vi "zwangstest.vi"() -> ()   [LabVIEW 2010]
panel:
  in  "Stopp 2":bool
  out "Zwangsbedingung!":dbl[](array[numeric])
  out "Zwangsbedingung?":bool[](array[boolean])
  in  "AbfragbVariablen":dbl[](array[numeric])
  out "Zwangsneurosen":string[][](array[string])
  in  "Bedingung Nr. X":i32
  in  "löschen":bool
  in  "Bedingung übernehmen":bool
  in  "Stopp":bool
  in  "Wert 2":dbl
  in  "Wert 1":dbl
  in  "Vergleichsoperator":dbl(ring) items=["<", "<=", "=", ">=", ">", "=/="]
  in  "BedienbareVariablen":dbl(ring) items=["Mod5/DIO0", "Mod5/DIO1", "Mod5/DIO2", "Mod5/DIO3", "Mod5/DIO4", "Mod5/DIO5", "Mod5/DIO6", "Mod5/DIO7", "Mod5/DIO8", "Mod5/DIO9", "Mod5/DIO10", "Mod5/DIO11", "Mod5/DIO12", "Mod5/DIO13", "Mod5/DIO14", "Mod5/DIO15", "Mod5/DIO16", "Mod5/DIO17", "Mod5/DIO18", "Mod5/DIO19", "Mod5/DIO20", "Mod5/DIO21", "Mod5/DIO22", "Mod5/DIO23", "Mod5/DIO24", "Mod5/DIO25", "Mod5/DIO26", "Mod5/DIO27", "Mod5/DIO28", "Mod5/DIO29", "Mod5/DIO30", "Mod5/DIO31", "Mod6/DIO0", "Mod6/DIO1", "Mod6/DIO2", "Mod6/DIO3", "Mod6/DIO4", "Mod6/DIO5", "Mod6/DIO6", "Mod6/DIO7", "Mod6/DIO8", "Mod6/DIO9", "Mod6/DIO10", "Mod6/DIO11", "Mod6/DIO12", "Mod6/DIO13", "Mod6/DIO14", "Mod6/DIO15", "Mod6/DIO16", "Mod6/DIO17", "Mod6/DIO18", "Mod6/DIO19", "Mod6/DIO20", "Mod6/DIO21", "Mod6/DIO22", "Mod6/DIO23", "Mod6/DIO24", "Mod6/DIO25", "Mod6/DIO26", "Mod6/DIO27", "Mod6/DIO28", "Mod6/DIO29", "Mod6/DIO30", "Mod6/DIO31", "ServoTrap1kalt", "ServoTrap2kalt", "Heizen?Trap1", "Heizen?Trap2", "Heizen?Mach1", "Heizen?Mach2", "LHHorst1Heizen?", "LHMainCol1Heizen?", "LHMainCol2Heizen?", "LHHorst2Heizen?", "LHOvenHeizen?", "LHT-LineHeizen?", "SPHorst1", "SPHorst2", "SPHorst3", "SPHorst4", "SPHorst5", "SPHorst6", "SPHorst7", "SPHorst8", "SPHorst9", "SPHorst10", "SPHorst11", "SPHorst12", "SPHorst13", "SPHorst14", "SPHorst15"]
  in  "AbfragbareVariablen":dbl(ring) items=["Mod1/AI0", "Mod1/AI1", "Mod1/AI2", "Mod1/AI3", "Mod1/AI4", "Mod1/AI5", "Mod1/AI6", "Mod1/AI7", "Mod1/AI8", "Mod1/AI9", "Mod1/AI10", "Mod1/AI11", "Mod1/AI12", "Mod1/AI13", "Mod1/AI14", "Mod1/AI15", "Mod1/AI16", "Mod1/AI17", "Mod1/AI18", "Mod1/AI19", "Mod1/AI20", "Mod1/AI21", "Mod1/AI22", "Mod1/AI23", "Mod1/AI24", "Mod1/AI25", "Mod1/AI26", "Mod1/AI27", "Mod1/AI28", "Mod1/AI29", "Mod1/AI30", "Mod1/AI31", "Mod2/AI0", "Mod2/AI1", "Mod2/AI2", "Mod2/AI3", "Mod2/AI4", "Mod2/AI5", "Mod2/AI6", "Mod2/AI7", "Mod2/AI8", "Mod2/AI9", "Mod2/AI10", "Mod2/AI11", "Mod2/AI12", "Mod2/AI13", "Mod2/AI14", "Mod2/AI15", "Mod2/AI16", "Mod2/AI17", "Mod2/AI18", "Mod2/AI19", "Mod2/AI20", "Mod2/AI21", "Mod2/AI22", "Mod2/AI23", "Mod2/AI24", "Mod2/AI25", "Mod2/AI26", "Mod2/AI27", "Mod2/AI28", "Mod2/AI29", "Mod2/AI30", "Mod2/AI31", "Mod3/AI0", "Mod3/AI1", "Mod3/AI2", "Mod3/AI3", "Mod3/AI4", "Mod3/AI5", "Mod3/AI6", "Mod3/AI7", "Mod3/AI8", "Mod3/AI9", "Mod3/AI10", "Mod3/AI11", "Mod3/AI12", "Mod3/AI13", "Mod3/AI14", "Mod3/AI15", "Mod3/AI16", "Mod3/AI17", "Mod3/AI18", "Mod3/AI19", "Mod3/AI20", "Mod3/AI21", "Mod3/AI22", "Mod3/AI23", "Mod3/AI24", "Mod3/AI25", "Mod3/AI26", "Mod3/AI27", "Mod3/AI28", "Mod3/AI29", "Mod3/AI30", "Mod3/AI31", "WiderstTrap1", "TempTrap1", "WiderstTrap2", "TempTrap2", "TempMach1", "TempMach2", "MWHorst1", "MWHorst2", "MWHorst3", "MWHorst4", "MWHorst5", "MWHorst6", "MWHorst7", "MWHorst8", "MWHorst9", "MWHorst10", "MWHorst11", "MWHorst12", "MWHorst13", "MWHorst14", "MWHorst15"]
  # "===>>"
  # "="
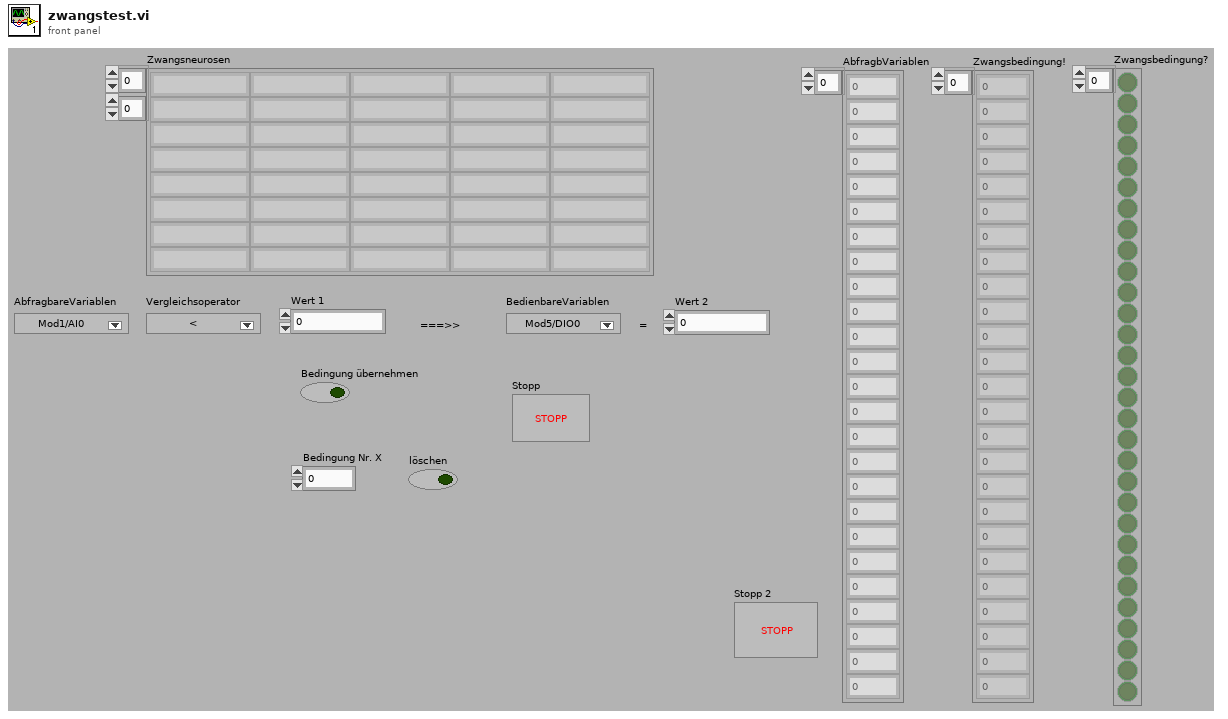
[diagram p1: front panel]
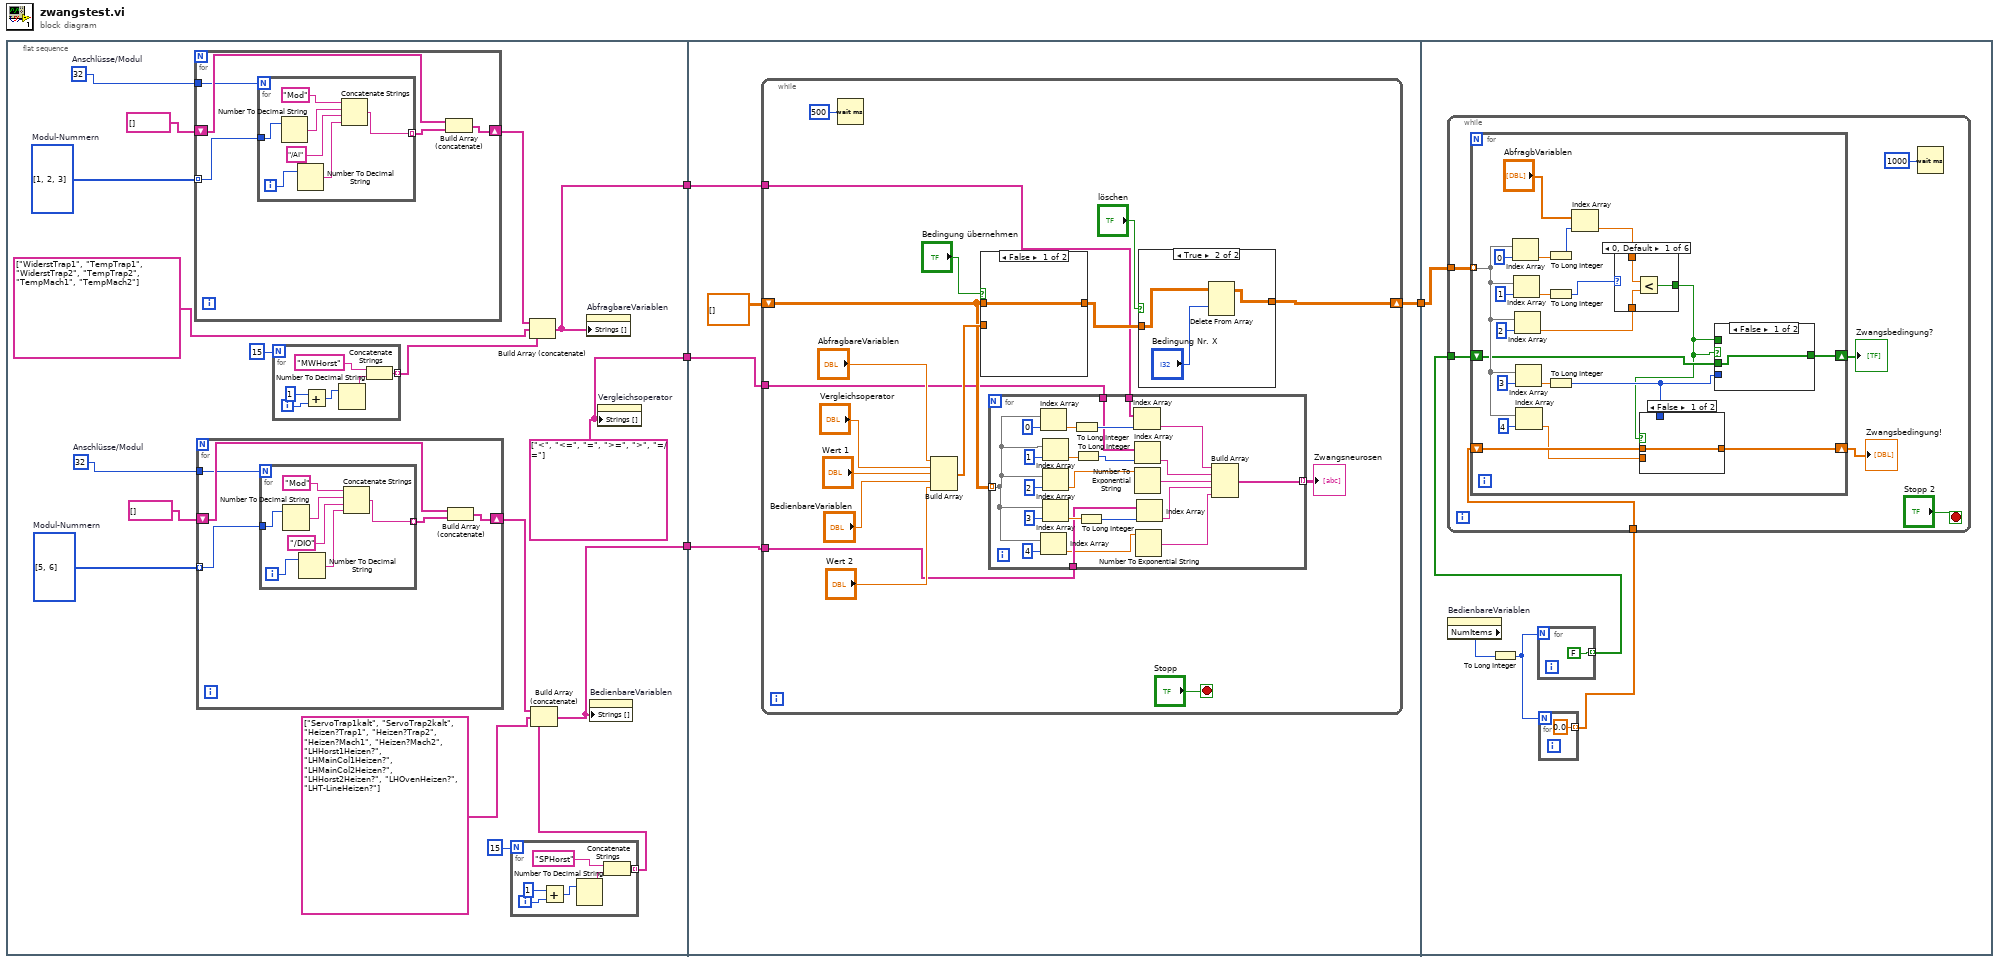
[diagram p0: block diagram]
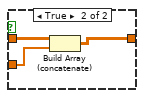
[diagram p3: hidden frame]
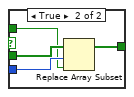
[diagram p4: hidden frame]
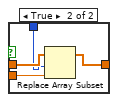
[diagram p5: hidden frame]
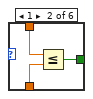
[diagram p6: hidden frame]
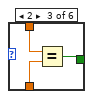
[diagram p7: hidden frame]
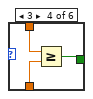
[diagram p8: hidden frame]
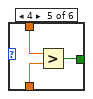
[diagram p9: hidden frame]
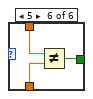
[diagram p10: hidden frame]
diagram:
  n1 = flat-sequence {
    tunnel: [w13] -> w4
    tunnel: [w12] -> w3
    tunnel: [w11] -> w2
    tunnel: w4 -> [w61]
    tunnel: w3 -> [w60]
    tunnel: w2 -> [w59]
    tunnel: [w58] -> w1
    tunnel: w1 -> [w112]
    frame #0 {
      w12 = string[] ["<", "<=", "=", ">=", ">", "=/="] ("Strings []")
      w16 = 32  # Anschlüsse/Modul
      w15 = i32[] [5, 6]  # Modul-Nummern
      w20 = 32  # Anschlüsse/Modul
      w19 = i32[] [1, 2, 3]  # Modul-Nummern
      n2 = for {
        shift-right: [w48] -> w21
        shift-left: string[] [] -> [w50]
        tunnel: w19 -> [w47] mode=indexing
        tunnel: w20 -> [w46]
        n3 = for {
          N: w46 -> [_]
          tunnel: [w56] -> w49 mode=indexing
          tunnel: w47 -> [w54]
          i -> [w57]
          n4 = Number To Decimal String(number=w54) -> (decimal integer string=w53:string)  [unwired: 1 in]
          n5 = Number To Decimal String(number=w57) -> (decimal integer string=w51:string)  [unwired: 1 in]
          n6 = Concatenate Strings("Mod", w53, "/AI", w51) -> (w56:string)
        }
        n7 = Build Array (concatenate)(w50, w49) -> (w48:string[])
      }
      n8 = for {
        shift-right: [w36] -> w17
        shift-left: string[] [] -> [w38]
        tunnel: w15 -> [w35] mode=indexing
        tunnel: w16 -> [w34]
        n9 = for {
          N: w34 -> [_]
          tunnel: [w44] -> w37 mode=indexing
          tunnel: w35 -> [w42]
          i -> [w45]
          n10 = Number To Decimal String(number=w42) -> (decimal integer string=w41:string)  [unwired: 1 in]
          n11 = Number To Decimal String(number=w45) -> (decimal integer string=w39:string)  [unwired: 1 in]
          n12 = Concatenate Strings("Mod", w41, "/DIO", w39) -> (w44:string)
        }
        n13 = Build Array (concatenate)(w38, w37) -> (w36:string[])
      }
      n14 = for {
        N: 15 -> [_]
        tunnel: [w28] -> w7 mode=indexing
        i -> [w33]
        n15 = Add(x=1, y=w33) -> (x+y=w31:i32)
        n16 = Number To Decimal String(number=w31) -> (decimal integer string=w29:string)  [unwired: 1 in]
        n17 = Concatenate Strings("MWHorst", w29) -> (w28:string)
      }
      n18 = for {
        N: 15 -> [_]
        tunnel: [w22] -> w5 mode=indexing
        i -> [w27]
        n19 = Add(x=1, y=w27) -> (x+y=w25:i32)
        n20 = Number To Decimal String(number=w25) -> (decimal integer string=w23:string)  [unwired: 1 in]
        n21 = Concatenate Strings("SPHorst", w23) -> (w22:string)
      }
      n22 = Build Array (concatenate)(w21, string[] ["WiderstTrap1", "TempTrap1", "WiderstTrap2", "TempTrap2", "TempMach1", "TempMach2"], w7) -> (w13:string[])
      n23 = Build Array (concatenate)(w17, string[] ["ServoTrap1kalt", "ServoTrap2kalt", "Heizen?Trap1", "Heizen?Trap2", "Heizen?Mach1", "Heizen?Mach2", "LHHorst1Heizen?", "LHMainCol1Heizen?", "LHMainCol2Heizen?", "LHHorst2Heizen?", "LHOvenHeizen?", "LHT-LineHeizen?"], w5) -> (w11:string[])
      n24 = property on="AbfragbareVariablen" class="Ring (strikt)"("Strings []"=w13) -> ()  [unwired: 2 in, 2 out]
      n25 = property on="BedienbareVariablen" class="Ring (strikt)"("Strings []"=w11) -> ()  [unwired: 2 in, 2 out]
      n26 = property on="Vergleichsoperator" class="Ring (strikt)"("Strings []"=w12) -> ()  [unwired: 2 in, 2 out]
    }
    frame #1 {
      n27 = while {
        shift-right: [w69] -> w58
        shift-left: dbl[][] [] -> [w67]
        tunnel: w61 -> [w66]
        tunnel: w60 -> [w65]
        tunnel: w59 -> [w64]
        stop <- "Stopp" stop-if-true
        n28 = Wait (ms)(milliseconds to wait=u32 500 ("Zu wartende ms")) -> ()  [unwired: 1 out]
        n29 = Build Array("AbfragbareVariablen", "Vergleichsoperator", "Wert 1", "BedienbareVariablen", "Wert 2") -> (w71:dbl[])
        n30 = case shown="False" "Bedingung übernehmen" {
          tunnel: w67 -> [w107 w110]
          tunnel: w71 -> [_ w109]
          tunnel: [w107 w108] -> w70
          frame False {
          }
          frame True {
            n31 = Build Array (concatenate)(w110, w109) -> (w108:dbl[][])
          }
        }
        n32 = for {
          tunnel: w67 -> [w102] mode=indexing
          tunnel: w66 -> [w90]
          tunnel: w65 -> [w89]
          tunnel: w64 -> [w88]
          tunnel: [w80] -> w63 mode=indexing
          n33 = Index Array(array=w102, index=0 ("Index")) -> (element=w96:dbl)
          n34 = Index Array(array=w102, index=4 ("Index")) -> (element=w86:dbl)
          n35 = Index Array(array=w102, index=1 ("Index")) -> (element=w94:dbl)
          n36 = Index Array(array=w102, index=2 ("Index")) -> (element=w87:dbl)
          n37 = Index Array(array=w102, index=3 ("Index")) -> (element=w92:dbl)
          n38 = To Long Integer(number=w96) -> (32bit integer=w95:i32)
          n39 = To Long Integer(number=w94) -> (32bit integer=w93:i32)
          n40 = To Long Integer(number=w92) -> (32bit integer=w91:i32)
          n41 = Index Array(array=w90, index=w95) -> (element=w85:string)
          n42 = Index Array(array=w89, index=w93) -> (element=w84:string)
          n43 = Number To Exponential String(number=w87) -> (E-format string=w83:string)  [unwired: 3 in]
          n44 = Number To Exponential String(number=w86) -> (E-format string=w81:string)  [unwired: 3 in]
          n45 = Index Array(array=w88, index=w91) -> (element=w82:string)
          n46 = Build Array(w85, w84, w83, w82, w81) -> (w80:string[])
        }
        "Zwangsneurosen" <- w63
        n47 = case shown="True" "löschen" {
          tunnel: w70 -> [w103 w106]
          tunnel: [w103 w104] -> w69
          frame False {
          }
          frame True {
            n48 = Delete From Array(array=w106, index (row)="Bedingung Nr. X") -> (array with subset deleted=w104:dbl[][])  [unwired: 2 in, 1 out]
          }
        }
      }
    }
    frame #2 {
      n49 = property on="BedienbareVariablen" class="Ring (strikt)"() -> ("NumItems"=w114:u32)  [unwired: 2 in, 2 out]
      n50 = To Long Integer(number=w114) -> (32bit integer=w113:i32)
      n51 = for {
        N: w113 -> [_]
        tunnel: [FALSE] -> w115 mode=indexing
      }
      n52 = for {
        N: w113 -> [_]
        tunnel: [0.0] -> w111 mode=indexing
      }
      n53 = while {
        tunnel: w112 -> [w123]
        tunnel: w115 -> [w122]
        tunnel: w111 -> [w118]
        stop <- "Stopp 2" stop-if-true
        n54 = for {
          tunnel: w123 -> [w131] mode=indexing
          shift-right: [w124] -> w120
          shift-left: w122 -> [w127]
          shift-right: [w128] -> w117
          shift-left: w118 -> [w130]
          n55 = Index Array(array=w131, index=0 ("Index")) -> (element=w142:dbl)
          n56 = Index Array(array=w131, index=1 ("Index")) -> (element=w140:dbl)
          n57 = Index Array(array=w131, index=2 ("Index")) -> (element=w136:dbl)
          n58 = Index Array(array=w131, index=3 ("Index")) -> (element=w133:dbl)
          n59 = Index Array(array=w131, index=4 ("Index")) -> (element=w129:dbl)
          n60 = To Long Integer(number=w142) -> (32bit integer=w135:i32)
          n61 = To Long Integer(number=w140) -> (32bit integer=w139:i32)
          n62 = To Long Integer(number=w133) -> (32bit integer=w126:i32)
          n63 = Index Array(array="AbfragbVariablen", index=w135) -> (element=w138:dbl)
          n64 = case shown="0, Default" w139 {
            tunnel: w138 -> [w157 w159 w163 w166 w169 w172]
            tunnel: w136 -> [w156 w160 w162 w165 w168 w171]
            tunnel: [w155 w158 w161 w164 w167 w170] -> w125
            frame 0, Default {
              n65 = Less?(x=w157, y=w156) -> (x < y?=w155:bool)
            }
            frame 1 {
              n66 = Less Or Equal?(x=w159, y=w160) -> (x <= y?=w158:bool)
            }
            frame 2 {
              n67 = Equal?(x=w163, y=w162) -> (x = y?=w161:bool)
            }
            frame 3 {
              n68 = Greater Or Equal?(x=w166, y=w165) -> (x >= y?=w164:bool)
            }
            frame 4 {
              n69 = Greater?(x=w169, y=w168) -> (0:w167:bool)
            }
            frame 5 {
              n70 = Not Equal?(x=w172, y=w171) -> (x != y?=w170:bool)
            }
          }
          n71 = case shown="False" w125 {
            tunnel: w130 -> [w150 w154]
            tunnel: w126 -> [_ w153]
            tunnel: w129 -> [_ w152]
            tunnel: [w150 w151] -> w128
            frame False {
            }
            frame True {
              n72 = Replace Array Subset(array=w154, new element=w152, index=w153) -> (w151:dbl[])
            }
          }
          n73 = case shown="False" w125 {
            tunnel: w127 -> [w145 w149]
            tunnel: w126 -> [_ w148]
            tunnel: w125 -> [_ w147]
            tunnel: [w145 w146] -> w124
            frame False {
            }
            frame True {
              n74 = Replace Array Subset(array=w149, new element=w147, index=w148) -> (w146:bool[])
            }
          }
        }
        "Zwangsbedingung?" <- w120
        "Zwangsbedingung!" <- w117
        n75 = Wait (ms)(milliseconds to wait=u32 1000 ("Zu wartende ms")) -> ()  [unwired: 1 out]
      }
    }
  }
